vi "close.vi"(8 "error in":errorcluster, 11 "MBParam in":refnum<class "MB Param.lvclass">) -> (0 "error out":errorcluster)   [LabVIEW 2021, in "MBParam.lvlib" / "MB Param.lvclass"]
uses:
  MB Param.lvclass
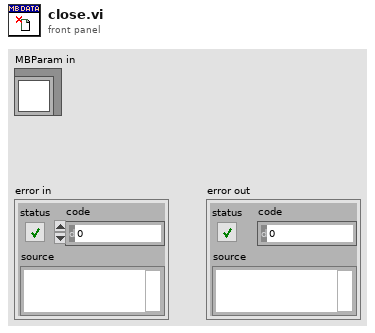
[diagram p1: front panel]
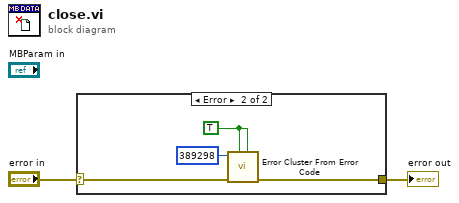
[diagram p0: block diagram]
diagram:
  n1 = case shown="Error" "error in" {
    selector: "error in" -> [w3 w7]
    tunnel: [w3 w6] -> w2
    frame No Error {
    }
    frame Error {
      w4 = TRUE ("show call chain? (False)")
      n2 = call <vilib>:"Error Cluster From Error Code.vi"("is warning? (False)"=w4, "show call chain? (False)"=w4, "error in (no error)"=w7, "error code (0)"=389298) -> ("error out"=w6:errorcluster)  [unwired: 5 in]
    }
  }
  "error out" <- w2
